vi "LotNoArray.vi"(10 "COMPNTSN":string, 11 "LotNo":string) -> (3 "COMPNTLOT":string)   [LabVIEW 2014]
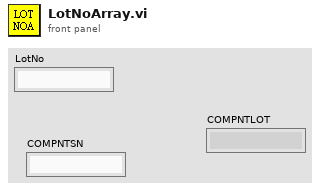
[diagram p1: front panel]
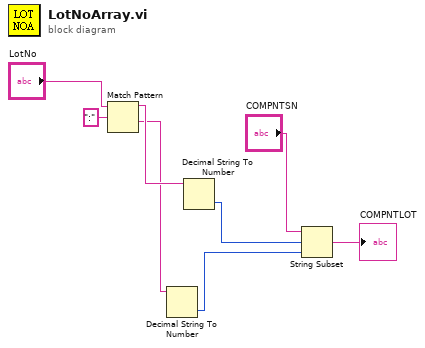
[diagram p0: block diagram]
diagram:
  n1 = Match Pattern(string="LotNo", regular expression=":") -> (before substring=w7:string, after substring=w6:string)  [unwired: 1 in, 2 out]
  n2 = Decimal String To Number(string=w6) -> (number=w4:i32)  [unwired: 2 in, 1 out]
  n3 = Decimal String To Number(string=w7) -> (number=w5:i32)  [unwired: 2 in, 1 out]
  n4 = String Subset(string="COMPNTSN", offset (0)=w5, length (rest)=w4) -> (substring=→"COMPNTLOT":string)
